vi "CheckDeviation.vi"(9 "CalSettings":T3={"SollPegel[dBSPL]"=94, "maxDeviationRef[dB]"=2.0, "maxDeviation[dB]"=2.0, "maxRuns"=20, "RefFrequency[Hz]"=94, "Wait[ms]"=0} {"maxDeviation[dB]" format="%.1f"; "maxDeviationRef[dB]" format="%.1f"}, 10 "Frequency List":T2(array[cluster]), 11 "fundamental amplitude":T4) -> (0 "error Out":errorcluster, 1 "DeviationInRange":bool, 2 "max value":dbl, 3 "min value":dbl, 5 "RefValue[dB]":dbl, 7 "output cluster":T1)   [LabVIEW 2018]
panel:
  out "RefAmp[V]":dbl
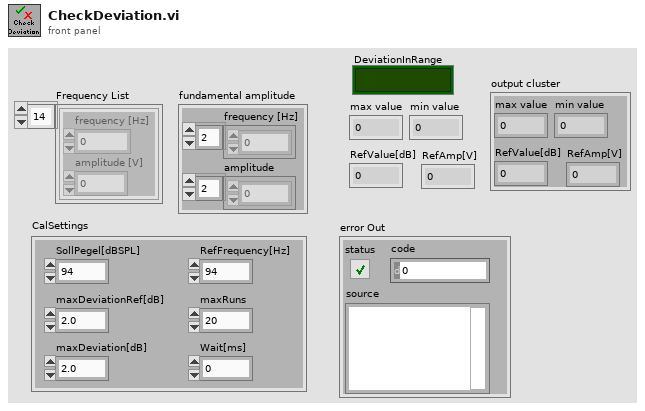
[diagram p1: front panel]
types:
  T1 = cluster{"max value":dbl, "min value":dbl, "RefValue[dB]":dbl, "RefAmp[V]":dbl}
  T2 = cluster{"frequency [Hz]":dbl, "amplitude [V]":dbl}[]
  T3 = cluster{"SollPegel[dBSPL]":i32, "maxDeviationRef[dB]":dbl, "maxDeviation[dB]":dbl, "maxRuns":i32, "RefFrequency[Hz]":i32, "Wait[ms]":i32}
  T4 = cluster{"frequency [Hz]":dbl[], "amplitude":dbl[]}
  T5 = cluster{"frequency [Hz]":dbl, "amplitude [V]":dbl}
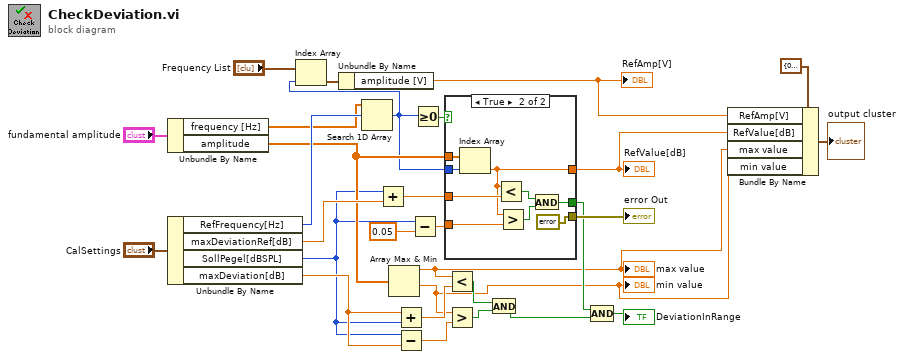
[diagram p0: block diagram]
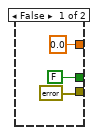
[diagram p2: hidden frame]
diagram:
  n1 = Unbundle By Name("fundamental amplitude") -> ("frequency [Hz]"=w19:dbl[], "amplitude"=w17:dbl[])
  n2 = Unbundle By Name("CalSettings") -> ("RefFrequency[Hz]"=w21:i32, "maxDeviationRef[dB]"=w22:dbl, "SollPegel[dBSPL]"=w11:i32, "maxDeviation[dB]"=w23:dbl)
  n3 = Search 1D Array(1D array=w19, element=w21) -> (index of element=w8:i32)  [unwired: 1 in]
  n4 = Index Array(array="Frequency List", index=w8) -> (element=w7:T5)
  n5 = Unbundle By Name(w7) -> ("amplitude [V]"=w2:dbl)
  "RefAmp[V]" <- w2
  n6 = Add(x=w11, y=w22) -> (x+y=w20:dbl)
  n7 = Array Max & Min(array=w17) -> (max value=w4:dbl, min value=w5:dbl)  [unwired: 2 out]
  "max value" <- w4
  "min value" <- w5
  n8 = Add(x=w23, y=w11) -> (x+y=w26:dbl)
  n9 = Subtract(x=w11, y=w23) -> (x-y=w25:dbl)
  n10 = Subtract(x=w11, y=0.05 ("x+y")) -> (x-y=w12:dbl)
  n11 = Greater Or Equal To 0?(x=w8) -> (x >= 0?=w18:bool)
  n12 = case shown="True" w18 {
    tunnel: w8 -> [_ w41]
    tunnel: w17 -> [_ w40]
    tunnel: w20 -> [_ w36]
    tunnel: w12 -> [_ w35]
    tunnel: [FALSE w37] -> w15
    tunnel: [0.0 ("element") w34] -> w3
    tunnel: [errorcluster {"status"=TRUE, "code"=-999, "source"="no Reference Frequency found"} ("error constant") errorcluster {"status"=FALSE, "code"=0, "source"=""} ("error constant")] -> w16
    frame False {
    }
    frame True {
      n13 = Index Array(array=w40, index=w41) -> (element=w34:dbl)
      n14 = Less?(x=w34, y=w36) -> (x < y?=w39:bool)
      n15 = Greater?(x=w34, y=w35) -> (0:w38:bool)
      n16 = And(x=w39, y=w38) -> (x .and. y?=w37:bool)
    }
  }
  "RefValue[dB]" <- w3
  "error Out" <- w16
  n17 = Less?(x=w4, y=w26) -> (x < y?=w28:bool)
  n18 = Greater?(x=w5, y=w25) -> (0:w27:bool)
  n19 = And(x=w28, y=w27) -> (x .and. y?=w14:bool)
  n20 = Compound Arithmetic op=AND(w15, w14) -> (→"DeviationInRange":bool)
  n21 = Bundle By Name(cluster=T1 {"max value"=0.0, "min value"=0.0, "RefValue[dB]"=0.0, "RefAmp[V]"=0.0} ("input cluster"), "RefAmp[V]"=w2, "RefValue[dB]"=w3, "max value"=w4, "min value"=w5) -> (→"output cluster":T1)
